vi "Remove Top Level Library.vi"(7 "error in":errorcluster, 10 "sourceItems":refnum<class "AB_Source.lvclass">[](array[class])) -> (0 "error out":errorcluster, 3 "sourceItems out":refnum<class "AB_Source.lvclass">[](array[class]))   [LabVIEW 2020, in "NI_AB_API_PPL.lvclass"]
uses:
  <vilib>/AppBuilder/AB_API/PPL/NI_AB_API_PPL.lvclass
  <vilib>/AppBuilder/AB_Classes/Source/AB_Source.lvclass
  <vilib>/AppBuilder/AB_Classes/Source/Library/AB_Source_Library.lvclass
  e:/builds/penguin/labview/branches/2020/dev/dist/vi.lib/AppBuilder/AB_Classes/Source/AB_Source.lvclass
  <vilib>/AppBuilder/AB_Source_Inclusion.ctl
  <vilib>/AppBuilder/AB_API/PPL/NI_AB_API_PPL.lvclass/NI_AB_API_PPL.ctl
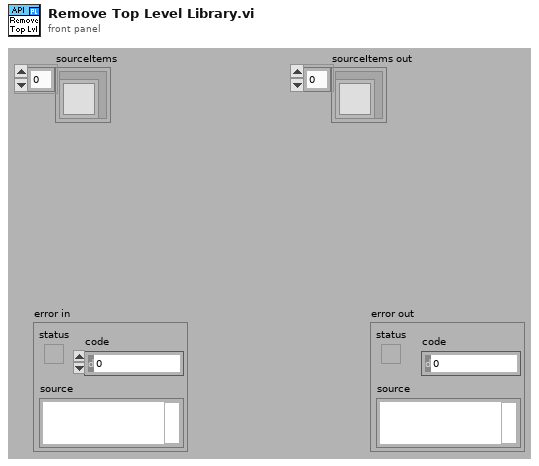
[diagram p1: front panel]
types:
  T1 = typedef "AB_Source_Inclusion.ctl" = enum16{"IncludeIfReferenced", "Include", "Exclude", "TopLevel"}
  T2 = typedef "AB_Source_Library.ctl" = cluster{"relinkCallers":bool, "atomicCopy":bool, "allowMissingMembers":bool, "eng_newDelimitedName":string, "eng_hasNonVILinks":bool, "eng_reference":refnum<vi>, "LVLIBPtopLevel":bool}
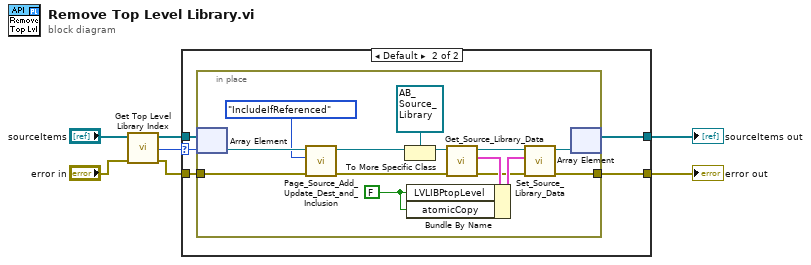
[diagram p0: block diagram]
diagram:
  n1 = call <vilib>:"Get Top Level Library Index.vi"("error in"="error in", "sourceItems"="sourceItems") -> ("error out"=w1:errorcluster, "Index"=w3:i32, "sourceItems out"=w7:refnum<class "AB_Source.lvclass">[])  [unwired: 7 in]
  n2 = case shown="Default" w3 {
    selector: w3 -> [_ w10]
    tunnel: w7 -> [w9 w14]
    tunnel: [w9 w13] -> w6
    tunnel: w1 -> [w8 w12]
    tunnel: [w8 w11] -> w4
    frame -1 {
    }
    frame Default {
      n3 = in-place {
        in-place-border: w12 -> [w27]
        in-place-border: [w19] -> w11
        w15 = FALSE ("LVLIBPtopLevel")
        n4 = in-place-array #1(w14, w10) -> (w28:refnum<class "AB_Source.lvclass">)
        n5 = call <vilib>:"Page_Source_Add_Update_Dest_and_Inclusion.vi"("error in (no error)"=w27, "Inclusion"=AB_Source_Inclusion."IncludeIfReferenced", "AB_Source_VI in"=w28) -> ("error out"=w18:errorcluster, "AB_Source_VI out"=w16:refnum<class "AB_Source.lvclass">)  [unwired: 1 in, 6 out]
        n6 = To More Specific Class(target class=refnum<class "AB_Source_Library.lvclass"> refnum ("AB_Source_Library.lvclass"), reference=w16) -> (specific class reference=w25:refnum<class "AB_Source_Library.lvclass">)  [unwired: 1 in, 1 out]
        n7 = call <vilib>:"Get_Source_Library_Data.vi"("error in (no error)"=w18, "Class in"=w25) -> ("error out"=w21:errorcluster, "data"=w22:T2, "Class out"=w24:refnum<class "AB_Source_Library.lvclass">)  [unwired: 7 in]
        n8 = Bundle By Name(cluster=w22, "LVLIBPtopLevel"=w15, "atomicCopy"=w15) -> (w23:T2)
        n9 = call <vilib>:"Set_Source_Library_Data.vi"("error in (no error)"=w21, "data"=w23, "Class in"=w24) -> ("error out"=w19:errorcluster, "Class out"=w20:refnum<class "AB_Source_Library.lvclass">)  [unwired: 7 in]
        n10 = in-place-array #1(w20) -> (w13:refnum<class "AB_Source.lvclass">[])  [unwired: 1 out]
      }
    }
  }
  "error out" <- w4
  "sourceItems out" <- w6
